vi "Get Multi OmniBus.vi"(8 "error in (no error)":errorcluster, 9 "Tag":string[](array[string]), 10 "Value Type":refnum<class "Omni_Bus.lvclass">[](array[class]), 11 "Var Bus in":refnum<class "Omni_Bus.lvclass">) -> (0 "error out":errorcluster, 1 "Updated Tags":bool[](array[boolean]), 2 "Value Out":refnum<class "Omni_Bus.lvclass">[](array[class]), 3 "Var Bus out":refnum<class "Omni_Bus.lvclass">)   [LabVIEW 2021, in "Omni_Bus.lvclass"]
uses:
  Omni_Bus.lvclass
  C:/Program Files (x86)/National Instruments/LabVIEW 2021/vi.lib/TSA/Abstract Data Classes/Abs_Types/Type/Abs_Type.lvclass
  <vilib>/TSA/Abstract Data Classes/Abs_Types/Type/Abs_Type.lvclass/Abs_Type.ctl
  Omni_Bus.lvclass/Omni_Bus.ctl
  FindVar.vi
  <vilib>/Utility/error.llb/Clear Errors.vi
  Properties/Read Var Map.vi
  <vilib>/TSA/Abstract Data Classes/Abs_Types/Type/Properties/Read Tag.vi
  <vilib>/TSA/Abstract Data Classes/Abs_Types/Value/Abs_Value.lvclass
  Check For Read Only Error.vi
  Incorrect Tag String Error.vi
  <vilib>/TSA/Abstract Data Classes/Abs_Types/Type/Abs_Type.lvclass
  C:/TSA/Omni-Bus/Source/Omni-Bus/Omni_Bus.lvclass
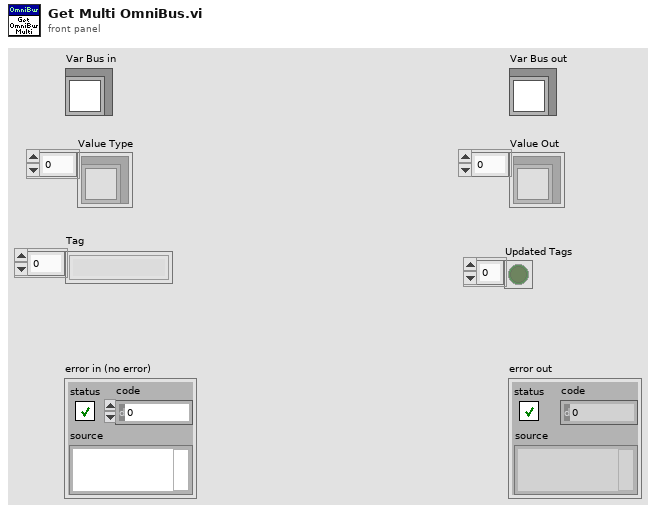
[diagram p1: front panel]
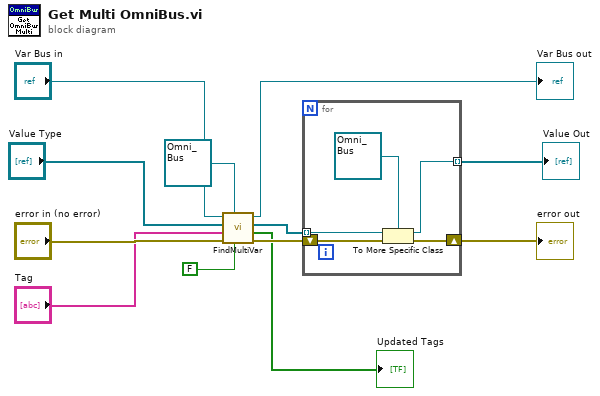
[diagram p0: block diagram]
diagram:
  n1 = call "FindMultiVar.vi"("Write?"=FALSE, "Abs_Type"=refnum<class "Omni_Bus.lvclass"> refnum ("Abs_Numeric.lvclass out"), "error in (no error)"="error in (no error)", "Tag"="Tag", "Abs_Type Default"="Value Type", "Var Bus in"="Var Bus in") -> ("error out"=w9:errorcluster, "Updated Tags"=→"Updated Tags":bool[], "Abs_Type Found"=w8:refnum<class "Abs_Type.lvclass">[], "Var Bus out"=→"Var Bus out":refnum<class "Omni_Bus.lvclass">)  [unwired: 2 in]
  n2 = for {
    tunnel: w8 -> [w16] mode=indexing
    tunnel: [w13] -> w4 mode=indexing
    shift-right: [w15] -> w6
    shift-left: w9 -> [w17]
    n3 = To More Specific Class(target class=refnum<class "Omni_Bus.lvclass"> refnum ("Abs_Numeric.lvclass out"), reference=w16, error in=w17) -> (specific class reference=w13:refnum<class "Omni_Bus.lvclass">, error out=w15:errorcluster)
  }
  "error out" <- w6
  "Value Out" <- w4
